vi "Split_path_all_sim.vi"() -> ()   [LabVIEW 2012]
panel:
  out "Path exists?":bool[](array[boolean])
  out "path type":i16[](array[numeric])
  out "path array":path[](array[path])
  in  "Path in":path
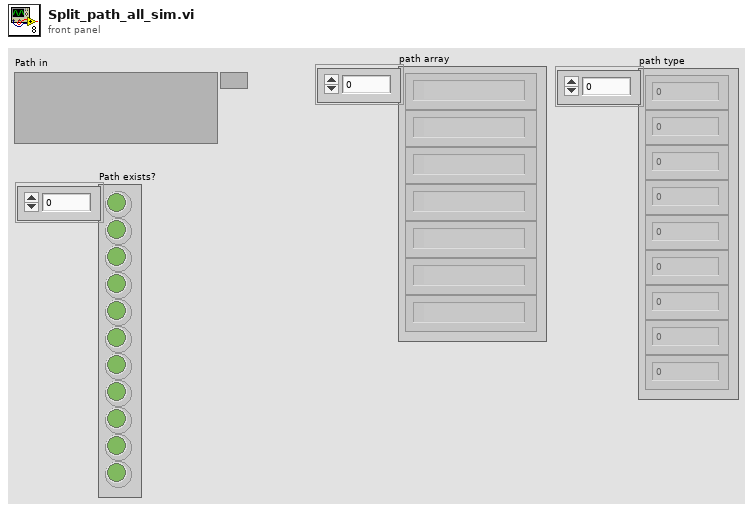
[diagram p1: front panel]
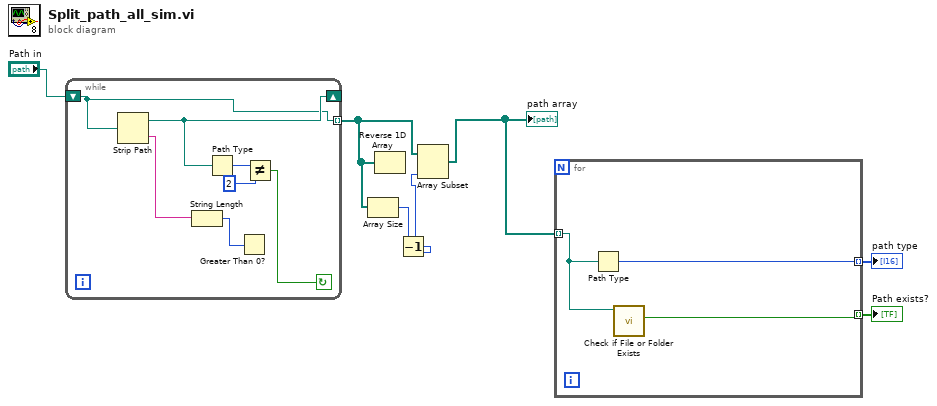
[diagram p0: block diagram]
diagram:
  n1 = while {
    tunnel: [w8] -> w2 mode=indexing
    shift-right: [w12] -> _
    shift-left: "Path in" -> [w8]
    stop <- w9 continue-if-true
    n2 = Strip Path(path=w8) -> (stripped path=w12:path, name=w14:string)
    n3 = String Length(string=w14) -> (length=w13:i32)
    n4 = Path Type(1:w12) -> (0:w11:i16)
    n5 = Greater Than 0?(x=w13) -> ()  [unwired: 1 out]
    n6 = Not Equal?(x=w11, y=i16 2) -> (x != y?=w9:bool)
  }
  n7 = Array Size(array=w2) -> (size(s)=w4:i32)
  n8 = Reverse 1D Array(array=w2) -> ()  [unwired: 1 out]
  n9 = Decrement(x=w4) -> (x-1=w3:i32)
  n10 = Array Subset(array=w2, length=w3) -> (w1:path[])  [unwired: 1 in]
  "path array" <- w1
  n11 = for {
    tunnel: w1 -> [w15] mode=indexing
    tunnel: [w17] -> w6 mode=indexing
    tunnel: [w16] -> w5 mode=indexing
    n12 = Path Type(1:w15) -> (0:w17:i16)
    n13 = call <vilib>:"Check if File or Folder Exists.vi"("path"=w15) -> ("file or folder exists?"=w16:bool)  [unwired: 8 in, 2 out]
  }
  "path type" <- w6
  "Path exists?" <- w5
